vi "Write to File.vi"(8 "error in":errorcluster, 10 "File Actor In":refnum<class "File Actor.lvclass">, 11 "Exe Write Main CMD in":refnum<class "Exe Write Main CMD.lvclass">) -> (0 "error out":errorcluster, 2 "File Actor Out":refnum<class "File Actor.lvclass">)   [LabVIEW 2016, in "Controller.lvlib" / "Exe Write Main CMD.lvclass"]
doc: "This is the sould of the execution method and the only VI that should be overriden. This is where we expect the file to be written."
uses:
  Exe Write Main CMD.lvclass
  File Actor/File Actor.lvclass
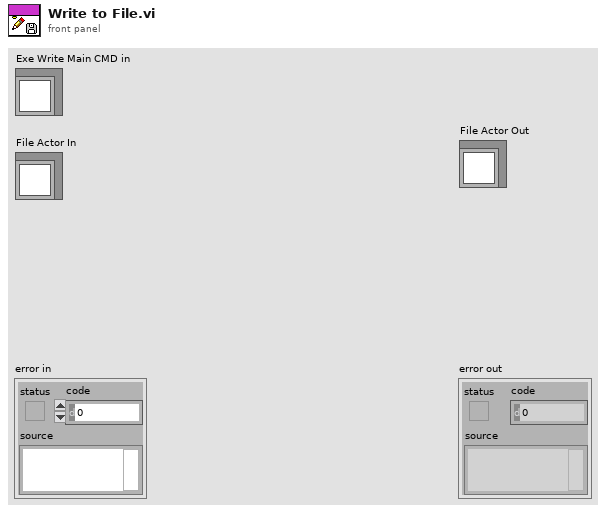
[diagram p1: front panel]
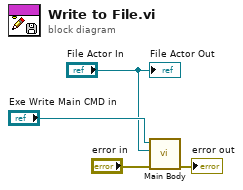
[diagram p0: block diagram]
diagram:
  n1 = call "Main Body.vi"("error in (no error)"="error in", "File Actor In"="File Actor In", "Exe Write Main CMD in"="Exe Write Main CMD in") -> ("error out"=→"error out":errorcluster)  [unwired: 8 in]
  "File Actor Out" <- "File Actor In"
